vi "Snapshot Example.vi"() -> ()   [LabVIEW 2020]
uses:
  g_industrial_cam/Device Enumeration.ctl
  g_industrial_cam/Camera/Camera.lvclass/Camera.ctl
  g_industrial_cam/Buffer/Buffer.lvclass/Buffer.ctl
  g_industrial_cam/Camera/GetSetPixelFormat.vi
  g_industrial_cam/Buffer/Create from Handle.vi
  g_industrial_cam/Buffer/GetBufferImageDimensions.vi
  g_industrial_cam/Camera/Check Not Disconnected.vi
  <vilib>/Utility/error.llb/Error Cluster From Error Code.vi
  <vilib>/picture/picture.llb/Draw 8-Bit Pixmap.vi
  g_industrial_cam/Buffer/Buffer.lvclass
  g_industrial_cam/Camera/Camera.lvclass
panel:
  out "Timeout":bool
  out "Devices":T1[](array[typedef])
  in  "Zoom":sgl caption="Picture Zoom Factor"
  out "Picture":picture
  out "Count":i32 caption="Snap Shot Count"
  in  "stop":bool
  out "error out":errorcluster
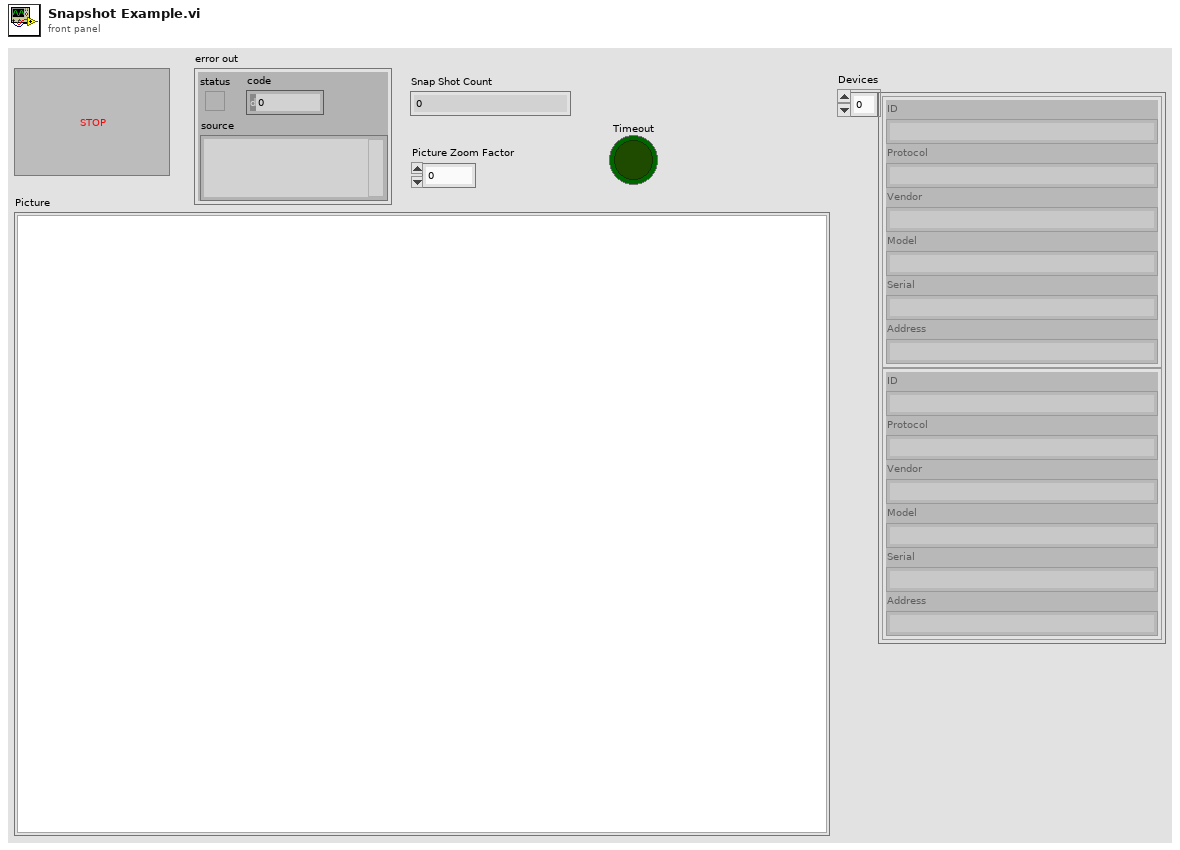
[diagram p1: front panel]
types:
  T1 = typedef "Device Enumeration.ctl" = cluster{"ID":string, "Protocol":string, "Vendor":string, "Model":string, "Serial":string, "Address":string}
  T2 = typedef "Buffer.lvclass/Image Size.ctl" = cluster{"Width":u16, "Height":u16}
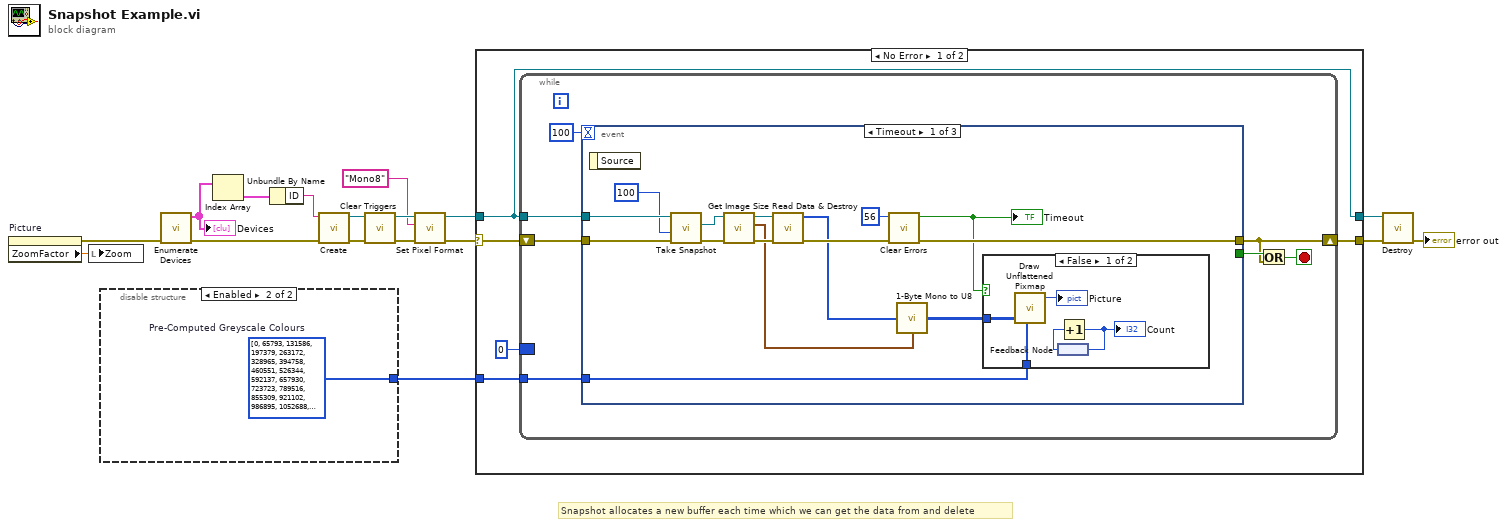
[diagram p0: block diagram]
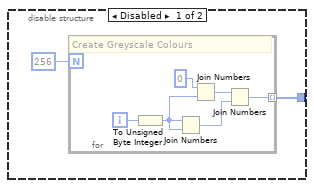
[diagram p2: hidden frame]
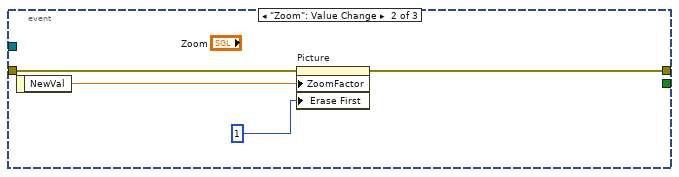
[diagram p4: hidden frame]
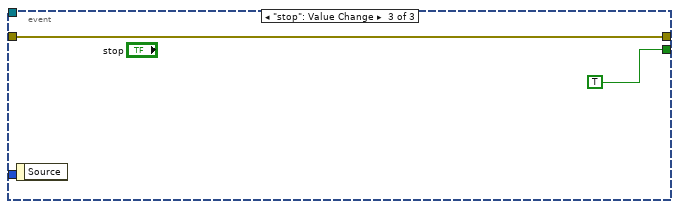
[diagram p5: hidden frame]
diagram:
  # "Snapshot allocates a new buffer each time which we can get the data from and delete"
  n1 = property on="Picture" class="Pict"() -> (error out=w8:errorcluster, "ZoomFactor"=w9:sgl)  [unwired: 2 in, 1 out]
  n2 = local write "Zoom"(w9) -> ()
  n3 = disable-structure shown="Enabled" {
    disable-tunnel: [w18 w26] -> w11
    frame Disabled {
      n4 = for {
        N: 256 -> [_]
        tunnel: [w20] -> w18 mode=indexing
        i -> [w25]
        # "Create Greyscale Colours"
        n5 = To Unsigned Byte Integer(number=w25) -> (unsigned 8bit integer=w24:u8)
        n6 = Join Numbers(hi=w24, lo=w24) -> ((hi.lo)=w21:u16)
        n7 = Join Numbers(hi=u8 0, lo=w24) -> ((hi.lo)=w22:u16)
        n8 = Join Numbers(hi=w22, lo=w21) -> ((hi.lo)=w20:u32)
      }
    }
    frame Enabled {
      w26 = u32[] [0, 65793, 131586, 197379, 263172, 328965, 394758, 460551, 526344, 592137, 657930, 723723, 789516, 855309, 921102, 986895, 1052688, 1118481, 1184274, 1250067, 1315860, 1381653, 1447446, 1513239, 1579032, 1644825, 1710618, 1776411, 1842204, 1907997, 1973790, 2039583, 2105376, 2171169, 2236962, 2302755, 2368548, 2434341, 2500134, 2565927, 2631720, 2697513, 2763306, 2829099, 2894892, 2960685, 3026478, 3092271, 3158064, 3223857, 3289650, 3355443, 3421236, 3487029, 3552822, 3618615, 3684408, 3750201, 3815994, 3881787, 3947580, 4013373, 4079166, 4144959, 4210752, 4276545, 4342338, 4408131, 4473924, 4539717, 4605510, 4671303, 4737096, 4802889, 4868682, 4934475, 5000268, 5066061, 5131854, 5197647, 5263440, 5329233, 5395026, 5460819, 5526612, 5592405, 5658198, 5723991, 5789784, 5855577, 5921370, 5987163, 6052956, 6118749, 6184542, 6250335, 6316128, 6381921, 6447714, 6513507, 6579300, 6645093, 6710886, 6776679, 6842472, 6908265, 6974058, 7039851, 7105644, 7171437, 7237230, 7303023, 7368816, 7434609, 7500402, 7566195, 7631988, 7697781, 7763574, 7829367, 7895160, 7960953, 8026746, 8092539, 8158332, 8224125, 8289918, 8355711, 8421504, 8487297, 8553090, 8618883, 8684676, 8750469, 8816262, 8882055, 8947848, 9013641, 9079434, 9145227, 9211020, 9276813, 9342606, 9408399, 9474192, 9539985, 9605778, 9671571, 9737364, 9803157, 9868950, 9934743, 10000536, 10066329, 10132122, 10197915, 10263708, 10329501, 10395294, 10461087, 10526880, 10592673, 10658466, 10724259, 10790052, 10855845, 10921638, 10987431, 11053224, 11119017, 11184810, 11250603, 11316396, 11382189, 11447982, 11513775, 11579568, 11645361, 11711154, 11776947, 11842740, 11908533, 11974326, 12040119, 12105912, 12171705, 12237498, 12303291, 12369084, 12434877, 12500670, 12566463, 12632256, 12698049, 12763842, 12829635, 12895428, 12961221, 13027014, 13092807, 13158600, 13224393, 13290186, 13355979, 13421772, 13487565, 13553358, 13619151, 13684944, 13750737, 13816530, 13882323, 13948116, 14013909, 14079702, 14145495, 14211288, 14277081, 14342874, 14408667, 14474460, 14540253, 14606046, 14671839, 14737632, 14803425, 14869218, 14935011, 15000804, 15066597, 15132390, 15198183, 15263976, 15329769, 15395562, 15461355, 15527148, 15592941, 15658734, 15724527, 15790320, 15856113, 15921906, 15987699, 16053492, 16119285, 16185078, 16250871, 16316664, 16382457, 16448250, 16514043, 16579836, 16645629, 16711422, 16777215]  # Pre-Computed Greyscale Colours
    }
  }
  n9 = call "Enumerate Devices.vi"("error in (no error)"=w8) -> ("error out"=w15:errorcluster, "Devices"=w17:T1[])  [unwired: 9 in]
  "Devices" <- w17
  n10 = Index Array(array=w17) -> (element=w16:T1)  [unwired: 1 in]
  n11 = Unbundle By Name(w16) -> ("ID"=w14:string)
  n12 = call "Create.vi"("error in (no error)"=w15, "Identifier (ID, IP etc)"=w14) -> ("error out"=w13:errorcluster, "Camera"=w10:refnum<class "Camera.lvclass">)  [unwired: 8 in]
  n13 = call "Clear Triggers.vi"("error in (no error)"=w13, "Camera in"=w10) -> ("error out"=w7:errorcluster, "Camera"=w4:refnum<class "Camera.lvclass">)  [unwired: 8 in]
  n14 = call "Set Pixel Format.vi"("error in (no error)"=w7, "Pixel Format"="Mono8", "Camera in"=w4) -> ("error out"=w2:errorcluster, "Camera"=w3:refnum<class "Camera.lvclass">)  [unwired: 7 in]
  n15 = case shown="No Error" w2 {
    selector: w2 -> [w31 w65]
    tunnel: w3 -> [w29 w66]
    tunnel: [w30 w65] -> w6
    tunnel: [w29 w66] -> w12
    tunnel: w11 -> [w28 _]
    frame No Error {
      n16 = while {
        shift-right: [w33] -> w30
        shift-left: w31 -> [w37]
        tunnel: w29 -> [w38]
        tunnel: w28 -> [w32]
        border: 0 -> [_]
        stop <- w34 stop-if-true
        n17 = event shown="[0] Timeout" {
          selector: _ -> [_ _ _]
          dyn-events: _ -> [_ _ _]
          timeout: 100 -> [_ _ _]
          tunnel: w38 -> [w53 _ _]
          tunnel: w37 -> [w52 w62 w64]
          tunnel: [w51 w61 w64] -> w33
          tunnel: [_ _ TRUE] -> w36
          tunnel: w32 -> [w50 _ _]
          event Timeout {
            n18 = event-data() -> ()  [unwired: 1 in, 1 out]
            n19 = call "Take Snapshot.vi"("error in (no error)"=w52, "Timeout (ms) (Default: 10000)"=100 ("Timeout (ms)"), "Camera in"=w53) -> ("error out"=w47:errorcluster, "New Buffer"=w48:refnum<class "Buffer.lvclass">)  [unwired: 6 in, 1 out]
            n20 = call "Get Image Size.vi"("error in (no error)"=w47, "Buffer in"=w48) -> ("error out"=w46:errorcluster, "Image Size"=w44:T2, "Buffer"=w45:refnum<class "Buffer.lvclass">)  [unwired: 7 in]
            n21 = call "Read Data & Destroy.vi"("error in (no error)"=w46, "Buffer in"=w45) -> ("error out"=w43:errorcluster, "Data"=w42:u8[])  [unwired: 8 in]
            n22 = call <vilib>:"Clear Errors.vi"("error in (no error)"=w43, "specific error code to clear (0: all)"=56) -> ("error out"=w51:errorcluster, "specific error cleared?"=w39:bool)  [unwired: 4 in]
            "Timeout" <- w39
            n23 = call "1-Byte Mono to U8.vi"("1-Byte Mono Data"=w42, "Image Size"=w44) -> ("U8 Pixels"=w41:u8[][])
            n24 = case shown="False" w39 {
              tunnel: w50 -> [w58 _]
              tunnel: w41 -> [w56 _]
              frame False {
                n25 = call-poly <vilib>:"Draw Unflattened Pixmap.vi"("data"=w56, "color table"=w58) -> ("new picture"=→"Picture":picture)  [unwired: 7 in]
                n26 = feedback #1() -> (w55:i32)
                n27 = Increment(x=w55) -> (x+1=w54:i32)
                "Count" <- w54
                n28 = feedback-in #1(w54) -> ()
              }
              frame True {
              }
            }
          }
          event "Zoom": Value Change {
            n29 = event-data() -> ("NewVal"=w60:sgl)  [unwired: 1 in]
            n30 = property on="Picture" class="Pict"(error in=w62, "ZoomFactor"=w60, "Erase First"=u8 1) -> (error out=w61:errorcluster)  [unwired: 1 in, 1 out]
          }
          event "stop": Value Change {
            n31 = event-data() -> ()  [unwired: 1 in, 1 out]
          }
        }
        n32 = Or(x=w36, y=w33) -> (x .or. y?=w34:bool)
      }
    }
    frame Error {
    }
  }
  n33 = call "Destroy.vi"("error in (no error)"=w6, "Camera in"=w12) -> ("error out"=→"error out":errorcluster)  [unwired: 9 in]
